vi "Main.vi"() -> (0 "error out":errorcluster)   [LabVIEW 2022 SP3, in "Test.lvlib"]
uses:
  Controller/Controller.lvclass
  C:/Program Files (x86)/National Instruments/LabVIEW 2022/vi.lib/ActorFramework/Actor/Actor.lvclass
  <vilib>/ActorFramework/Message Enqueuer/Message Enqueuer.lvclass/Message Enqueuer.ctl
  <vilib>/ActorFramework/Message Enqueuer/Enqueue.vi
  <vilib>/ActorFramework/Stop Msg/Stop Msg.lvclass
  C:/Program Files (x86)/National Instruments/LabVIEW 2022/vi.lib/ActorFramework/Message/Message.lvclass
  <vilib>/ActorFramework/Message Priority Queue/Priority Enqueue.vi
  Test.lvlib
  <vilib>/ActorFramework/Actor/Actor.lvclass
  C:/Users/jakub/repos/gh/sw4sys/lv-logging-actor/LoggingActor/Source/LoggingActor/LoggingActor/LoggingActor.lvclass
  C:/Users/jakub/repos/gh/sw4sys/lv-logging-actor/LoggingActor/Source/Test/Controller/Controller.lvclass
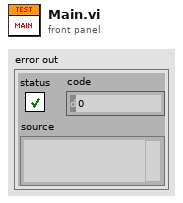
[diagram p1: front panel]
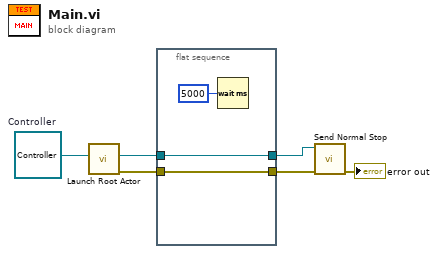
[diagram p0: block diagram]
diagram:
  w6 = refnum<class "Controller.lvclass"> refnum  # Controller
  n1 = call <vilib>:"Launch Root Actor.vi"("Actor"=w6) -> ("error out"=w4:errorcluster, "Actor's Enqueuer"=w5:refnum<class "Message Enqueuer.lvclass">)  [unwired: 9 in]
  n2 = flat-sequence {
    tunnel: w5 -> [w8]
    tunnel: w4 -> [w7]
    tunnel: [w8] -> w3
    tunnel: [w7] -> w2
    frame #0 {
      n3 = Wait (ms)(milliseconds to wait=u32 5000) -> ()  [unwired: 1 out]
    }
  }
  n4 = call <vilib>:"Send Normal Stop.vi"("error in (no error)"=w2, "Message Enqueuer"=w3) -> ("error out"=→"error out":errorcluster)  [unwired: 9 in]
